vi "Calculate Compass Vertices.vi"(6 "2D Compass Property":T1, 8 "error in (no error)":errorcluster, 9 "Vertex Cluster":T2, 11 "Polar Area Ref In":refnum<vi>) -> (0 "error out":errorcluster, 1 "Compass Vertex":cluster{"X":i16, "Y":i16}[][](array[cluster]), 3 "Polar Area Ref Out":refnum<vi>)   [LabVIEW 2020, in "2D Compass.lvclass"]
uses:
  <vilib>/Math Plots/2D Math Plots/2D Compass/2D Compass/2D Compass.lvclass
  <vilib>/Math Plots/2D Math Plots/2D Compass/2D Compass/Typedef/2D Compass Property.ctl
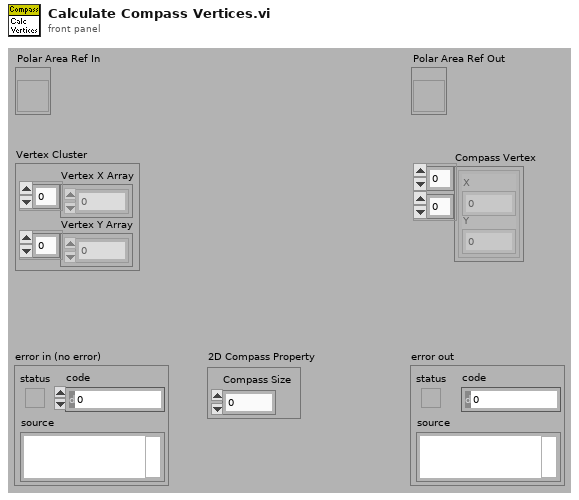
[diagram p1: front panel]
types:
  T1 = typedef "2D Compass.lvclass/2D Compass Property.ctl" = cluster{"Compass Size":dbl}
  T2 = cluster{"Vertex X Array":dbl[], "Vertex Y Array":dbl[]}
  T3 = typedef "LVPoint32TypeDef.ctl" = cluster{"Horizontal":i32, "Vertical":i32}
  T4 = typedef "LVRectTypeDef.ctl" = cluster{"left":i16, "top":i16, "right":i16, "bottom":i16}
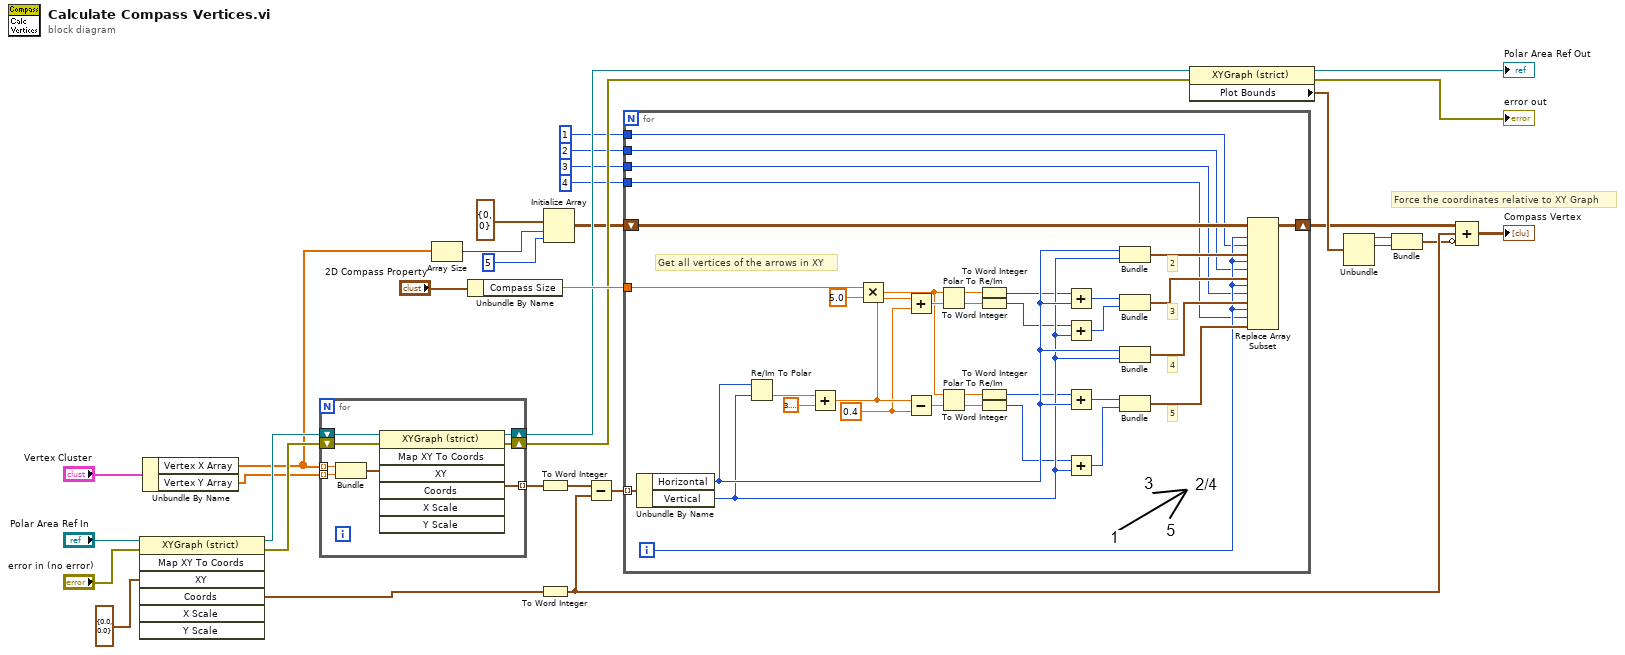
[diagram p0: block diagram]
diagram:
  # "Force the coordinates relative to XY Graph"
  n1 = invoke class="XYGraph (strict)" method="Map XY To Coords"(reference="Polar Area Ref In", error in="error in (no error)", "XY"=cluster{"X":dbl, "Y":dbl} {"X"=0.0, "Y"=0.0}) -> (reference out=w23:refnum<vi>, error out=w19:errorcluster, "Coords"=w15:T3)  [unwired: 4 in, 4 out]
  n2 = Unbundle By Name("Vertex Cluster") -> ("Vertex X Array"=w9:dbl[], "Vertex Y Array"=w5:dbl[])
  n3 = for {
    tunnel: w9 -> [w41] mode=indexing
    tunnel: w5 -> [w40] mode=indexing
    tunnel: [w37] -> w17 mode=indexing
    shift-right: [w36] -> w21
    shift-left: w23 -> [w38]
    shift-right: [w34] -> w18
    shift-left: w19 -> [w35]
    n4 = Bundle("X"=w41, "X"=w40) -> (w39:cluster{"X":dbl, "X":dbl})  [unwired: 1 out]
    n5 = invoke class="XYGraph (strict)" method="Map XY To Coords"(reference=w38, error in=w35, "XY"=w39) -> (reference out=w36:refnum<vi>, error out=w34:errorcluster, "Coords"=w37:T3)  [unwired: 4 in, 4 out]
  }
  n6 = Array Size(array=w9) -> (size(s)=w7:i32)
  n7 = Unbundle By Name("2D Compass Property") -> ("Compass Size"=w31:dbl)
  n8 = To Word Integer(number=w17) -> (16bit integer=w14:cluster{"Horizontal":i16, "Vertical":i16}[])
  n9 = To Word Integer(number=w15) -> (16bit integer=w13:cluster{"Horizontal":i16, "Vertical":i16})
  n10 = Initialize Array(cluster{"X":i16, "Y":i16} {"X"=0, "Y"=0} ("XY"), w7, 5 ("dimension size")) -> (w8:cluster{"X":i16, "Y":i16}[][])
  n11 = Subtract(x=w14, y=w13) -> (x-y=w16:cluster{"Horizontal":i16, "Vertical":i16}[])
  n12 = for {
    tunnel: w31 -> [w65]
    tunnel: w16 -> [w58] mode=indexing
    shift-right: [w51] -> w12
    shift-left: w8 -> [w52]
    tunnel: 1 ("disabled index (row)") -> [w45]
    tunnel: 2 ("disabled index (row)") -> [w44]
    tunnel: 3 ("disabled index (row)") -> [w43]
    tunnel: 4 ("disabled index (row)") -> [w42]
    i -> [w46]
    w67 = 0.4 ("y")
    # "Get all vertices of the arrows in XY"
    # "5"
    # "4"
    # "3"
    # "2"
    n13 = Unbundle By Name(w58) -> ("Horizontal"=w60:i16, "Vertical"=w59:i16)
    n14 = Re/Im To Polar(2:w59, 3:w60) -> (0:w68:dbl)  [unwired: 1 out]
    n15 = Add(x=w68, y=3.141592653589793) -> (x+y=w69:dbl)
    n16 = Multiply(x=w65, y=5.0) -> (x*y=w66:dbl)
    n17 = Add(x=w69, y=w67) -> (x+y=w74:dbl)
    n18 = Subtract(x=w69, y=w67) -> (x-y=w75:dbl)
    n19 = Polar To Re/Im(2:w74, 3:w66) -> (0:w71:dbl, 1:w73:dbl)
    n20 = Polar To Re/Im(2:w75, 3:w66) -> (0:w70:dbl, 1:w72:dbl)
    n21 = To Word Integer(number=w73) -> (16bit integer=w56:i16)
    n22 = To Word Integer(number=w71) -> (16bit integer=w55:i16)
    n23 = To Word Integer(number=w72) -> (16bit integer=w54:i16)
    n24 = To Word Integer(number=w70) -> (16bit integer=w53:i16)
    n25 = Add(x=w56, y=w60) -> (x+y=w64:i16)
    n26 = Add(x=w55, y=w59) -> (x+y=w61:i16)
    n27 = Add(x=w54, y=w60) -> (x+y=w63:i16)
    n28 = Add(x=w53, y=w59) -> (x+y=w62:i16)
    n29 = Bundle("Horizontal"=w60, "Vertical"=w59) -> (w50:cluster{"Horizontal":i16, "Vertical":i16})  [unwired: 1 out]
    n30 = Bundle(w64, w61) -> (w49:cluster{i16, i16})  [unwired: 1 out]
    n31 = Bundle("Horizontal"=w60, "Vertical"=w59) -> (w48:cluster{"Horizontal":i16, "Vertical":i16})  [unwired: 1 out]
    n32 = Bundle(w63, w62) -> (w47:cluster{i16, i16})  [unwired: 1 out]
    n33 = Replace Array Subset(array=w52, new element #1=w50, index (row) #1=w46, index (col) #1=w45, new element #2=w49, index (row) #2=w46, index (col) #2=w44, new element #3=w48, index (row) #3=w46, index (col) #3=w43, new element #4=w47, index (row) #4=w46, index (col) #4=w42) -> (w51:cluster{"X":i16, "Y":i16}[][])
  }
  n34 = property class="XYGraph (strict)"(reference=w21, error in=w18) -> (reference out=→"Polar Area Ref Out":refnum<vi>, error out=→"error out":errorcluster, "Plot Bounds"=w27:T4)
  n35 = Unbundle(w27) -> ("left"=w29:i16, "top"=w28:i16)  [unwired: 2 out]
  n36 = Bundle("left"=w29, "top"=w28) -> (w11:cluster{"left":i16, "top":i16})  [unwired: 1 out]
  n37 = Compound Arithmetic op=ADD(w12, w13, invert w11) -> (→"Compass Vertex":cluster{i16, i16}[][])
